vi "File.Close.vi"(8 "error in":errorcluster, 11 "File ref in":refnum<file>) -> (0 "error out":errorcluster)   [LabVIEW 2016]
doc: "Writes to a file.\nIf <B>append</B> is false (default), the file will be rewritten.\nIf <B>append</B> is true, the new data will be appended to the file.\nSupports a <B>header</B> line which will be placed on top of the file when it is created or rewritten. This <B>header</B> line requires a newline at the end."
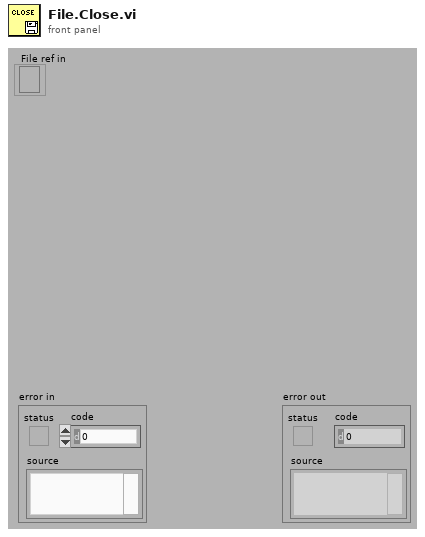
[diagram p1: front panel]
types:
  T1 = enum16{"deny read/write", "deny write-only", "deny none"}
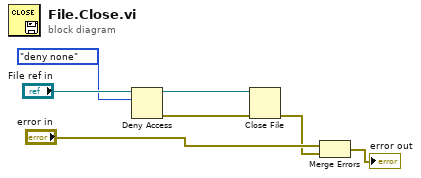
[diagram p0: block diagram]
diagram:
  n1 = Deny Access(6:T1."deny none" ("deny mode (0:deny read/write)"), 7:"File ref in") -> (0:w3:errorcluster, 3:w2:refnum<file>)  [unwired: 1 in]
  n2 = Close File(refnum=w2, error in=w3) -> (error out=w6:errorcluster)  [unwired: 1 out]
  n3 = Merge Errors("error in", w6) -> (→"error out":errorcluster)
